vi "Set Active Module.vi"(8 "error in (no error)":errorcluster, 11 "SLL Subpanel Manager in":refnum<class "SLL Subpanel Manager.lvclass">) -> (0 "error out":errorcluster, 3 "SLL Subpanel Manager out":refnum<class "SLL Subpanel Manager.lvclass">)   [LabVIEW 2014, in "SLL Subpanel Manager.lvclass"]
uses:
  SLL Subpanel Manager.lvclass
panel:
  in  "Module Name":string
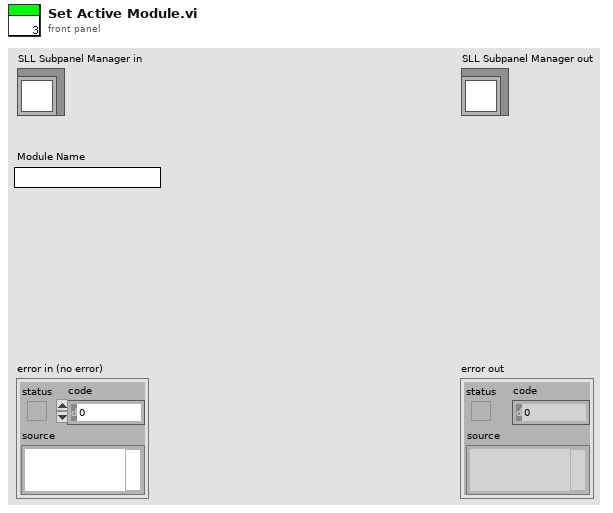
[diagram p1: front panel]
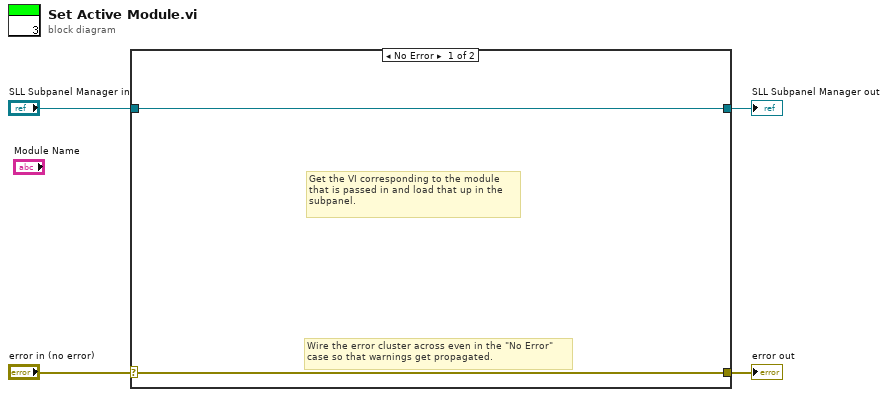
[diagram p0: block diagram]
diagram:
  n1 = case shown="No Error" "error in (no error)" {
    selector: "error in (no error)" -> [w5 w8]
    tunnel: [w5 w8] -> w3
    tunnel: [w6 w7] -> w1
    tunnel: "SLL Subpanel Manager in" -> [w6 w7]
    frame No Error {
      # "Get the VI corresponding to the module\nthat is passed in and load that up in the \nsubpanel."
      # "Wire the error cluster across even in the \"No Error\"\ncase so that warnings get propagated."
    }
    frame Error {
    }
  }
  "error out" <- w3
  "SLL Subpanel Manager out" <- w1
